vi "Ramp_BackForth_SubVI.vi"(6 "Enum":enum16{"Forward", "Backward"}(ring), 8 "index":i32, 9 "step":dbl, 10 "min":dbl, 11 "max":dbl) -> (0 "Stop?":bool, 1 "Numeric":dbl)   [LabVIEW 2010]
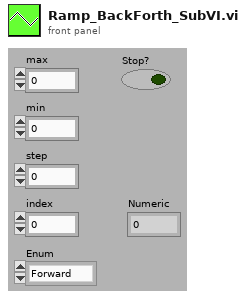
[diagram p1: front panel]
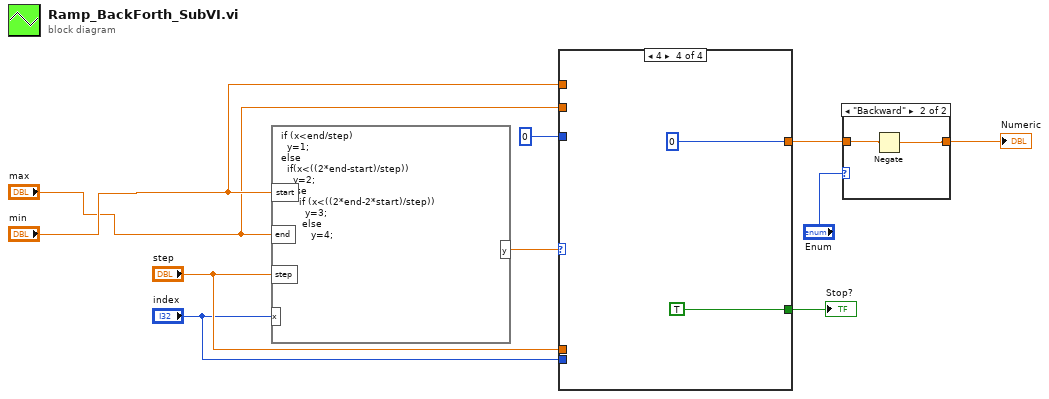
[diagram p0: block diagram]
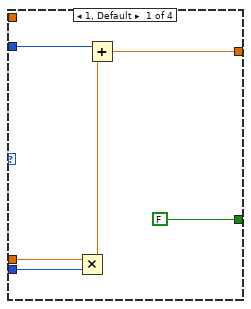
[diagram p3: hidden frame]
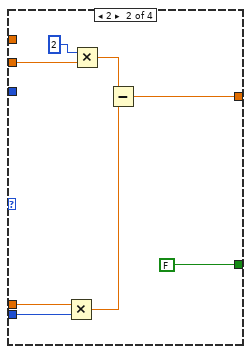
[diagram p4: hidden frame]
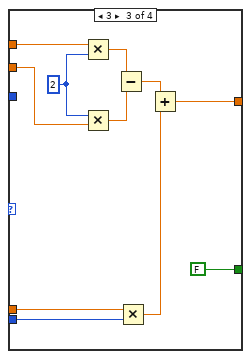
[diagram p5: hidden frame]
diagram:
  n1 = formula code="if (x<end/step)\n  y=1;\nelse\n  if(x<((2*end-start)/step))     \n    y=2;\n  else\n      if (x<((2*end-2*start)/step))\n        y=3;\n       else \n          y=4;"("x"="index", "start"="min", "end"="max", "step"="step") -> ("y"=w10:dbl)
  n2 = case shown="4" w10 {
    tunnel: 0 -> [w16 _ _ _]
    tunnel: "step" -> [w15 w22 w31 _]
    tunnel: "index" -> [w14 w21 w30 _]
    tunnel: [w12 w18 w27 0] -> w2
    tunnel: "max" -> [_ w24 w25 _]
    tunnel: "min" -> [_ _ w35 _]
    tunnel: [FALSE FALSE FALSE TRUE] -> w6
    frame 1, Default {
      n3 = Multiply(x=w15, y=w14) -> (x*y=w13:dbl)
      n4 = Add(x=w16, y=w13) -> (x+y=w12:dbl)
    }
    frame 2 {
      n5 = Multiply(x=w22, y=w21) -> (x*y=w19:dbl)
      n6 = Multiply(x=2, y=w24) -> (x*y=w20:dbl)
      n7 = Subtract(x=w20, y=w19) -> (x-y=w18:dbl)
    }
    frame 3 {
      w34 = 2
      n8 = Multiply(x=w35, y=w34) -> (x*y=w33:dbl)
      n9 = Multiply(x=w34, y=w25) -> (x*y=w32:dbl)
      n10 = Subtract(x=w33, y=w32) -> (x-y=w28:dbl)
      n11 = Multiply(x=w31, y=w30) -> (x*y=w29:dbl)
      n12 = Add(x=w28, y=w29) -> (x+y=w27:dbl)
    }
    frame 4 {
    }
  }
  "Stop?" <- w6
  n13 = case shown="\"Backward\"" "Enum" {
    tunnel: w2 -> [w38 w40]
    tunnel: [w38 w39] -> w1
    frame "Forward", Default {
    }
    frame "Backward" {
      n14 = Negate(x=w40) -> (-x=w39:dbl)
    }
  }
  "Numeric" <- w1
